vi "DoubleArray2StringArray.vi"(1 "Precision":string="%.8f", 2 "Double Array Input":dbl[](array[numeric])) -> (0 "STring Array Output":string[][](array[string]))   [LabVIEW 2019]
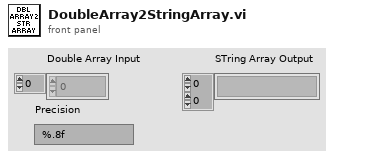
[diagram p1: front panel]
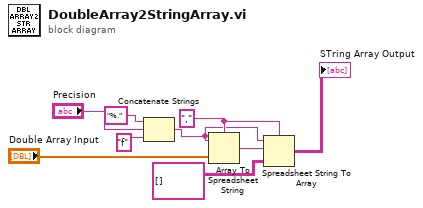
[diagram p0: block diagram]
diagram:
  w7 = "," ("delimiter (Tab)")
  n1 = Concatenate Strings("%." ("string"), "Precision", "f" ("string")) -> (w1:string)
  n2 = Array To Spreadsheet String(delimiter (Tab)=w7, array="Double Array Input", 3:w1) -> (spreadsheet string=w6:string)
  n3 = Spreadsheet String To Array(delimiter (Tab)=w7, format string=w1, spreadsheet string=w6, array type (2D Dbl)=string[][] []) -> (array=→"STring Array Output":string[][])
